vi "Main.vi"() -> ()   [LabVIEW 2022 SP3]
uses:
  Controls/MainStates.ctl
  <userlib>/_OpenG.lib/array/array.llb/Remove Duplicates from 1D Array (String)__ogtk.vi
panel:
  in  "Clean after \"(\"":bool
  out "New":string
  out "Old":string
  out "new path":path
  in  "Auto":enum32{"Manual", "MKV", "AVI", "MP4", "MP3"}(radio)
  in  "Commit":bool
  in  "Replacement String":string
  in  "Split Key":string="("
  in  "Method":T1(ring)
  in  "Extension":string=".*"
  in  "Path":path
  out "New":i32(listbox)
  out "Current":i32(listbox)=1
  in  "Exit":bool
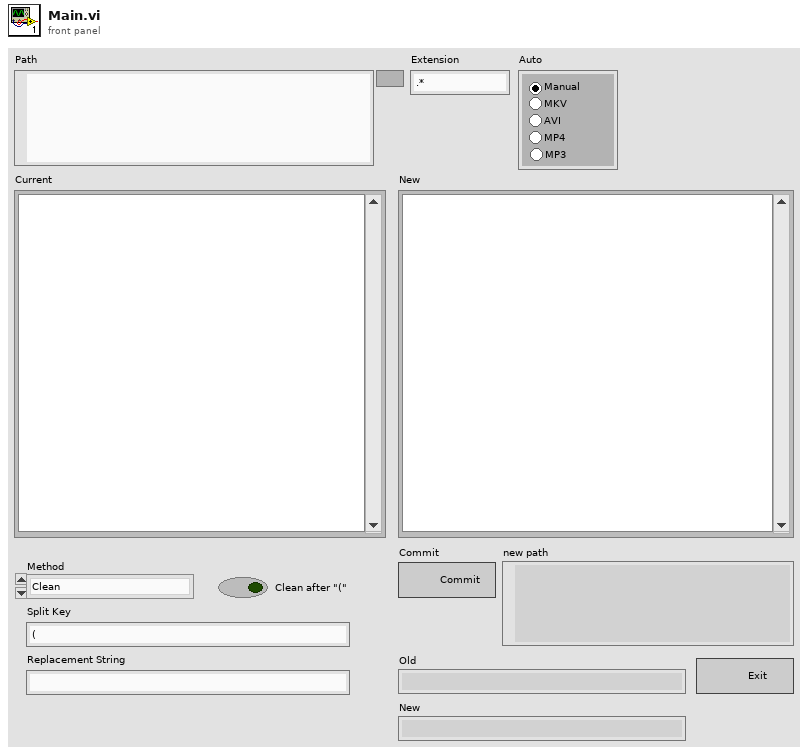
[diagram p1: front panel]
types:
  T1 = enum16{"Clean", "Replace", "Clear Periods", "Strip Prefix", "Add Prefix"}
  T2 = typedef "MainStates.ctl" = enum16{"Init", "Get Path", "Get Files", "Set Extension", "Check for Dups", "Clean", "Add Prefix", "Replace", "Periods", "Strip Prefix", "Commit", "Wait for Input", "Exit"}
  T3 = enum8{"Enabled", "Disabled", "Disabled and Grayed Out"}
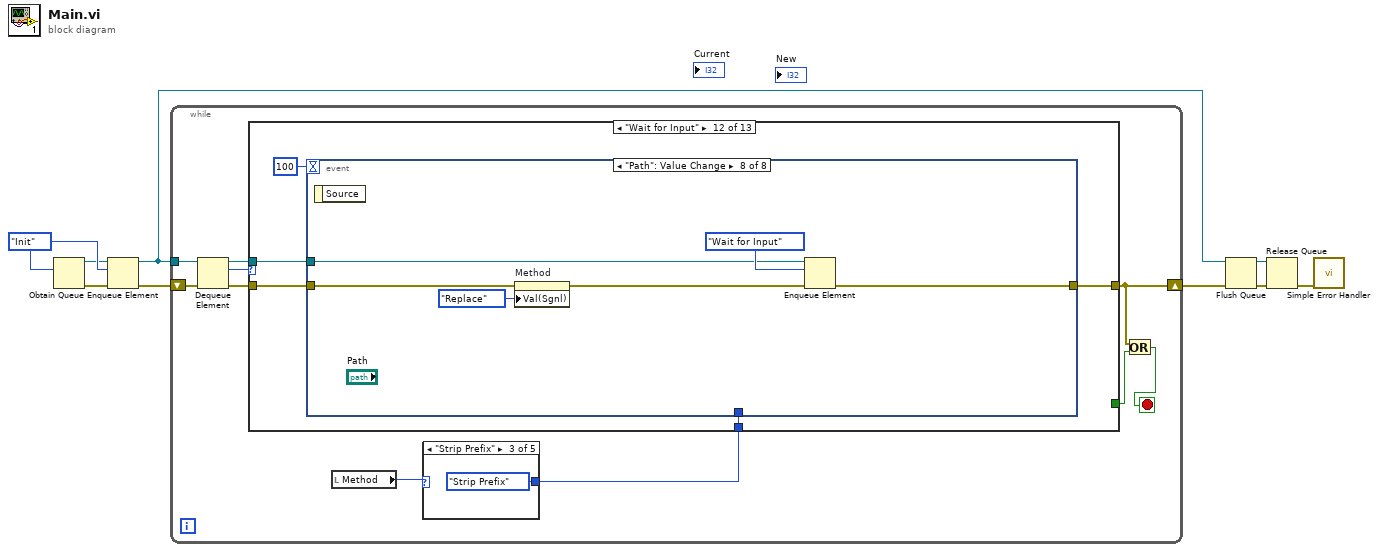
[diagram p0: block diagram]
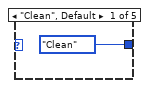
[diagram p2: hidden frame]
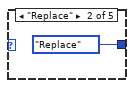
[diagram p3: hidden frame]
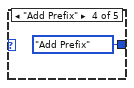
[diagram p4: hidden frame]
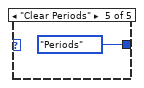
[diagram p5: hidden frame]
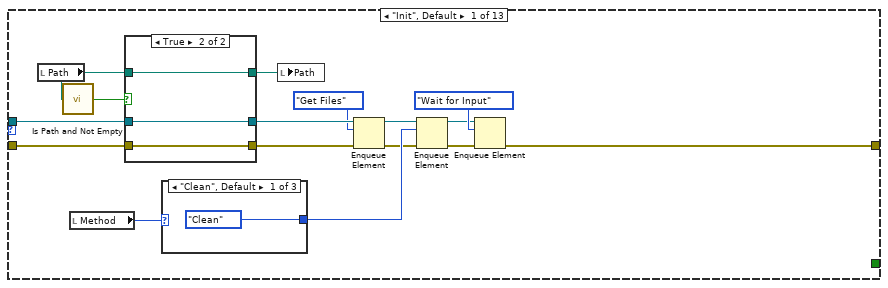
[diagram p6: hidden frame]
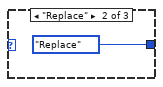
[diagram p7: hidden frame]
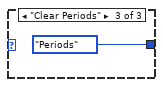
[diagram p8: hidden frame]
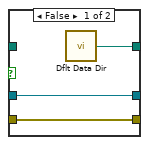
[diagram p9: hidden frame]
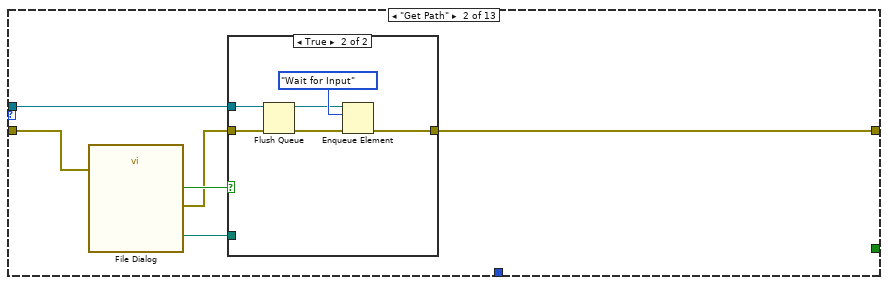
[diagram p10: hidden frame]
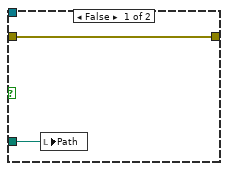
[diagram p11: hidden frame]
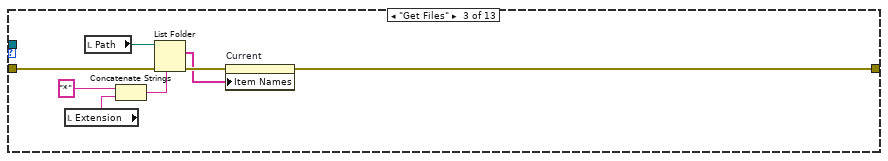
[diagram p12: hidden frame]
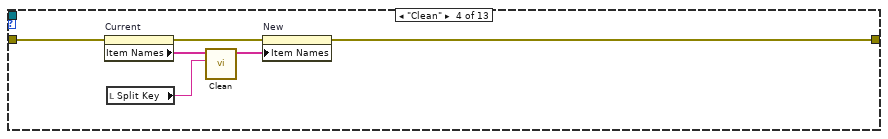
[diagram p13: hidden frame]
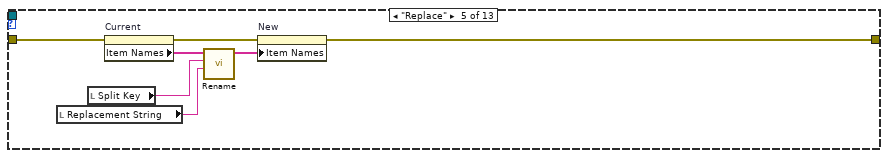
[diagram p14: hidden frame]
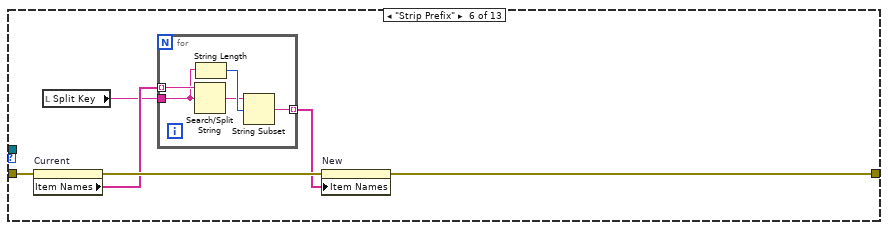
[diagram p15: hidden frame]
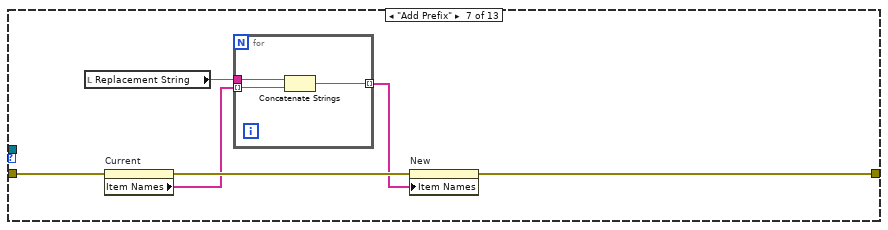
[diagram p16: hidden frame]
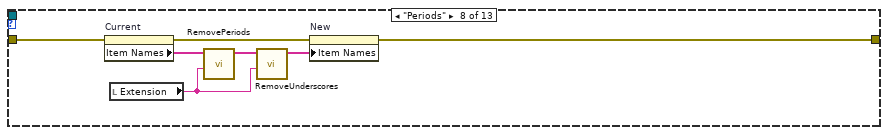
[diagram p17: hidden frame]
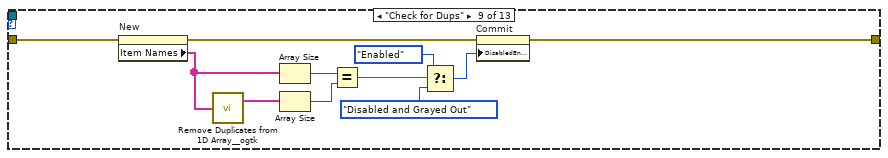
[diagram p18: hidden frame]
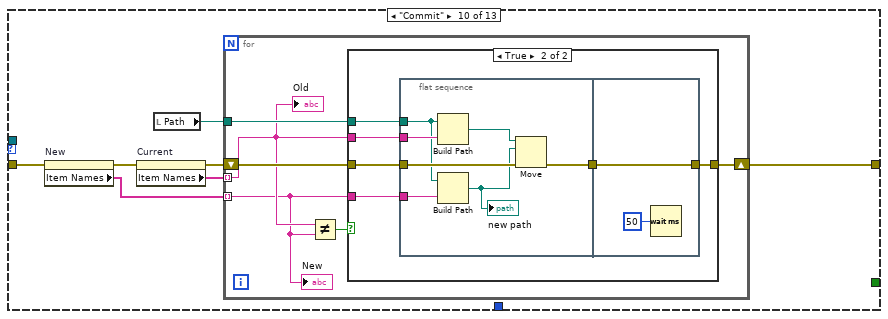
[diagram p19: hidden frame]
diagram:
  w9 = MainStates."Init" ("Main States")
  n1 = Obtain Queue(element data type=w9) -> (queue out=w8:refnum<queue>, error out=w7:errorcluster)  [unwired: 4 in, 1 out]
  n2 = Enqueue Element(queue=w8, element=w9, error in (no error)=w7) -> (queue out=w4:refnum<queue>, error out=w6:errorcluster)  [unwired: 1 in, 1 out]
  n3 = while {
    tunnel: w4 -> [w18]
    shift-right: [w12] -> w3
    shift-left: w6 -> [w19]
    stop <- w10 stop-if-true
    n4 = Dequeue Element(queue=w18, error in (no error)=w19) -> (queue out=w16:refnum<queue>, element=w17:T2, error out=w15:errorcluster)  [unwired: 1 in, 1 out]
    n5 = local read "Method"() -> (w14:T1)
    n6 = case shown="\"Strip Prefix\"" w14 {
      tunnel: [MainStates."Clean" ("Main States") MainStates."Replace" ("Main States") MainStates."Strip Prefix" ("Main States") MainStates."Add Prefix" ("Main States") MainStates."Periods" ("Main States")] -> w13
      frame "Clean", Default {
      }
      frame "Replace" {
      }
      frame "Strip Prefix" {
      }
      frame "Add Prefix" {
      }
      frame "Clear Periods" {
      }
    }
    n7 = case shown="\"Wait for Input\"" w17 {
      tunnel: w16 -> [w36 w53 _ _ _ _ _ _ _ _ _ w165 _]
      tunnel: w15 -> [w37 w55 w70 w77 w84 w90 w101 w111 w122 w127 w154 w164 w238]
      tunnel: [w39 w51 w64 w72 w78 w88 w99 w108 w115 w123 w152 w163 w238] -> w12
      tunnel: [_ _ _ _ _ _ _ _ _ _ _ _ TRUE] -> w11
      tunnel: w13 -> [_ _ _ _ _ _ _ _ _ _ _ w162 _]
      frame "Init", Default {
        n8 = local read "Path"() -> (w26:path)
        n9 = call <vilib>:"Is Path and Not Empty.vi"("path"=w26) -> ("Is Path and Not Empty?"=w38:bool)  [unwired: 4 in]
        n10 = local read "Method"() -> (w33:T1)
        n11 = case shown="True" w38 {
          tunnel: w37 -> [w45 w48]
          tunnel: w36 -> [w46 w49]
          tunnel: [w46 w49] -> w35
          tunnel: [w45 w48] -> w34
          tunnel: w26 -> [_ w47]
          tunnel: [w44 w47] -> w25
          frame False {
            n12 = call <vilib>:"Dflt Data Dir.vi"() -> ("App:Default Data Directory"=w44:path)
          }
          frame True {
          }
        }
        n13 = case shown="\"Clean\", Default" w33 {
          tunnel: [MainStates."Clean" ("Main States") MainStates."Replace" ("Main States") MainStates."Periods" ("Main States")] -> w30
          frame "Clean", Default {
          }
          frame "Replace" {
          }
          frame "Clear Periods" {
          }
        }
        n14 = local write "Path"(w25) -> ()
        n15 = Enqueue Element(queue=w35, element=MainStates."Get Files" ("Main States"), error in (no error)=w34) -> (queue out=w28:refnum<queue>, error out=w27:errorcluster)  [unwired: 1 in, 1 out]
        n16 = Enqueue Element(queue=w28, element=w30, error in (no error)=w27) -> (queue out=w31:refnum<queue>, error out=w32:errorcluster)  [unwired: 1 in, 1 out]
        n17 = Enqueue Element(queue=w31, element=MainStates."Wait for Input" ("Main States"), error in (no error)=w32) -> (error out=w39:errorcluster)  [unwired: 1 in, 2 out]
      }
      frame "Get Path" {
        n18 = call "File Dialog"("error in"=w55) -> ("selected path"=w50:path, "cancelled"=w54:bool, "error out"=w52:errorcluster)  [unwired: 11 in, 1 out]
        n19 = case shown="True" w54 {
          tunnel: w53 -> [_ w63]
          tunnel: w52 -> [w56 w62]
          tunnel: [w56 w58] -> w51
          tunnel: w50 -> [w57 _]
          frame False {
            n20 = local write "Path"(w57) -> ()
          }
          frame True {
            n21 = Flush Queue(queue=w63, error in (no error)=w62) -> (queue out=w60:refnum<queue>, error out=w59:errorcluster)  [unwired: 1 out]
            n22 = Enqueue Element(queue=w60, element=MainStates."Wait for Input" ("Main States"), error in (no error)=w59) -> (error out=w58:errorcluster)  [unwired: 1 in, 2 out]
          }
        }
      }
      frame "Get Files" {
        n23 = local read "Extension"() -> (w65:string)
        n24 = local read "Path"() -> (w71:path)
        n25 = Concatenate Strings("*", w65) -> (w66:string)
        n26 = List Folder(path=w71, pattern=w66, error in=w70) -> (filenames=w68:string[], error out=w69:errorcluster)  [unwired: 1 in, 2 out]
        n27 = property on="Current" class="LstBox (strict)"(error in=w69, "Item Names"=w68) -> (error out=w64:errorcluster)  [unwired: 1 in, 1 out]
      }
      frame "Clean" {
        n28 = property on="Current" class="LstBox (strict)"(error in=w77) -> (error out=w73:errorcluster, "Item Names"=w76:string[])  [unwired: 1 in, 1 out]
        n29 = local read "Split Key"() -> (w75:string)
        n30 = call "Clean.vi"("Split Key"=w75, "Filenames In"=w76) -> ("Filenames Out"=w74:string[])  [unwired: 9 in]
        n31 = property on="New" class="LstBox (strict)"(error in=w73, "Item Names"=w74) -> (error out=w72:errorcluster)  [unwired: 1 in, 1 out]
      }
      frame "Replace" {
        n32 = local read "Replacement String"() -> (w81:string)
        n33 = local read "Split Key"() -> (w82:string)
        n34 = property on="Current" class="LstBox (strict)"(error in=w84) -> (error out=w79:errorcluster, "Item Names"=w83:string[])  [unwired: 1 in, 1 out]
        n35 = call "Rename.vi"("Replacement String"=w81, "Split Key"=w82, "Filenames In"=w83) -> ("Filenames Out"=w80:string[])  [unwired: 8 in]
        n36 = property on="New" class="LstBox (strict)"(error in=w79, "Item Names"=w80) -> (error out=w78:errorcluster)  [unwired: 1 in, 1 out]
      }
      frame "Strip Prefix" {
        n37 = property on="Current" class="LstBox (strict)"(error in=w90) -> (error out=w89:errorcluster, "Item Names"=w87:string[])  [unwired: 1 in, 1 out]
        n38 = local read "Split Key"() -> (w86:string)
        n39 = for {
          tunnel: w87 -> [w95] mode=indexing
          tunnel: w86 -> [w94]
          tunnel: [w91] -> w85 mode=indexing
          n40 = Search/Split String(string=w95, search string/char (-)=w94) -> (match + rest of string=w92:string)  [unwired: 1 in, 2 out]
          n41 = String Length(string=w94) -> (length=w93:i32)
          n42 = String Subset(string=w92, offset (0)=w93) -> (substring=w91:string)  [unwired: 1 in]
        }
        n43 = property on="New" class="LstBox (strict)"(error in=w89, "Item Names"=w85) -> (error out=w88:errorcluster)  [unwired: 1 in, 1 out]
      }
      frame "Add Prefix" {
        n44 = local read "Replacement String"() -> (w97:string)
        n45 = property on="Current" class="LstBox (strict)"(error in=w101) -> (error out=w100:errorcluster, "Item Names"=w98:string[])  [unwired: 1 in, 1 out]
        n46 = for {
          tunnel: w98 -> [w104] mode=indexing
          tunnel: w97 -> [w103]
          tunnel: [w102] -> w96 mode=indexing
          n47 = Concatenate Strings(w103, w104) -> (w102:string)
        }
        n48 = property on="New" class="LstBox (strict)"(error in=w100, "Item Names"=w96) -> (error out=w99:errorcluster)  [unwired: 1 in, 1 out]
      }
      frame "Periods" {
        n49 = property on="Current" class="LstBox (strict)"(error in=w111) -> (error out=w109:errorcluster, "Item Names"=w110:string[])  [unwired: 1 in, 1 out]
        n50 = local read "Extension"() -> (w105:string)
        n51 = call "RemovePeriods.vi"("Extension"=w105, "Filenames In"=w110) -> ("Filenames Out"=w107:string[])  [unwired: 9 in]
        n52 = call "RemoveUnderscores.vi"("Extension"=w105, "Filenames In"=w107) -> ("Filenames Out"=w106:string[])  [unwired: 9 in]
        n53 = property on="New" class="LstBox (strict)"(error in=w109, "Item Names"=w106) -> (error out=w108:errorcluster)  [unwired: 1 in, 1 out]
      }
      frame "Check for Dups" {
        n54 = property on="New" class="LstBox (strict)"(error in=w122) -> (error out=w116:errorcluster, "Item Names"=w121:string[])  [unwired: 1 in, 1 out]
        n55 = call-poly <userlib>:"Remove Duplicates from 1D Array__ogtk.vi"("Input Array"=w121) -> ("Output Array"=w120:string[])  [unwired: 1 out]
        n56 = Array Size(array=w121) -> (size(s)=w119:i32)
        n57 = Array Size(array=w120) -> (size(s)=w118:i32)
        n58 = Equal?(x=w119, y=w118) -> (x = y?=w117:bool)
        n59 = Select(t=T3."Enabled" ("Disabled"), s=w117, f=T3."Disabled and Grayed Out" ("Disabled")) -> (s? t:f=w112:T3)
        n60 = property on="Commit" class="Bool"(error in=w116, "DisabledEnum"=w112) -> (error out=w115:errorcluster)  [unwired: 1 in, 1 out]
      }
      frame "Commit" {
        n61 = property on="New" class="LstBox (strict)"(error in=w127) -> (error out=w126:errorcluster, "Item Names"=w125:string[])  [unwired: 1 in, 1 out]
        n62 = property on="Current" class="LstBox (strict)"(error in=w126) -> (error out=w124:errorcluster, "Item Names"=w128:string[])  [unwired: 1 in, 1 out]
        n63 = local read "Path"() -> (w129:path)
        n64 = for {
          tunnel: w129 -> [w134]
          tunnel: w128 -> [w131] mode=indexing
          tunnel: w125 -> [w130] mode=indexing
          shift-right: [w133] -> w123
          shift-left: w124 -> [w135]
          n65 = Not Equal?(x=w131, y=w130) -> (x != y?=w132:bool)
          n66 = case shown="True" w132 {
            tunnel: w131 -> [_ w142]
            tunnel: w135 -> [w136 w141]
            tunnel: w134 -> [_ w140]
            tunnel: w130 -> [_ w139]
            tunnel: [w136 w138] -> w133
            frame False {
            }
            frame True {
              n67 = flat-sequence {
                tunnel: w142 -> [w149]
                tunnel: w141 -> [w148]
                tunnel: w140 -> [w147]
                tunnel: w139 -> [w146]
                tunnel: [w143] -> w137
                tunnel: [w151] -> w138
                tunnel: w137 -> [w151]
                frame #0 {
                  n68 = Build Path(base path=w147, name or relative path=w149) -> (appended path=w145:path)
                  n69 = Build Path(base path=w147, name or relative path=w146) -> (appended path=w144:path)
                  "new path" <- w144
                  n70 = Move(source path=w145, error in=w148, 10:w144) -> (error out=w143:errorcluster)  [unwired: 2 in, 2 out]
                }
                frame #1 {
                  n71 = Wait (ms)(milliseconds to wait=u32 50) -> ()  [unwired: 1 out]
                }
              }
            }
          }
          "Old" <- w131
          "New" <- w130
        }
      }
      frame "Set Extension" {
        n72 = local read "Auto"() -> (w155:enum32{"Manual", "MKV", "AVI", "MP4", "MP3"})
        n73 = case shown="\"MP3\"" w155 {
          tunnel: [".*" ".mkv" ".avi" ".mp4" ".mp3"] -> w153
          frame "Manual", Default {
          }
          frame "MKV" {
          }
          frame "AVI" {
          }
          frame "MP4" {
          }
          frame "MP3" {
          }
        }
        n74 = property on="Extension" class="Str"(error in=w154, "Val(Sgnl)"=w153) -> (error out=w152:errorcluster)  [unwired: 1 in, 1 out]
      }
      frame "Wait for Input" {
        n75 = event shown="[7] \"Path\": Value Change" {
          selector: _ -> [_ _ _ _ _ _ _ _]
          dyn-events: _ -> [_ _ _ _ _ _ _ _]
          timeout: 100 -> [_ _ _ _ _ _ _ _]
          tunnel: w165 -> [w169 w181 w188 w204 w217 w225 w229 w235]
          tunnel: w164 -> [w168 w180 w189 w205 w216 w223 w228 w234]
          tunnel: [w167 w178 w183 w197 w214 w219 w230 w236] -> w163
          tunnel: w162 -> [_ w177 _ w196 w212 _ _ _]
          event "Exit": Value Change {
            n76 = event-data() -> ()  [unwired: 1 in, 1 out]
            n77 = Enqueue Element(queue=w169, element=MainStates."Exit" ("Main States"), error in (no error)=w168) -> (error out=w167:errorcluster)  [unwired: 1 in, 2 out]
          }
          event Timeout {
            n78 = event-data() -> ()  [unwired: 1 in, 3 out]
            n79 = Enqueue Element(queue=w181, element=MainStates."Get Files" ("Main States"), error in (no error)=w180) -> (queue out=w175:refnum<queue>, error out=w174:errorcluster)  [unwired: 1 in, 1 out]
            n80 = Enqueue Element(queue=w175, element=w177, error in (no error)=w174) -> (queue out=w173:refnum<queue>, error out=w172:errorcluster)  [unwired: 1 in, 1 out]
            n81 = Enqueue Element(queue=w173, element=MainStates."Check for Dups" ("Main States"), error in (no error)=w172) -> (queue out=w171:refnum<queue>, error out=w170:errorcluster)  [unwired: 1 in, 1 out]
            n82 = Enqueue Element(queue=w171, element=MainStates."Wait for Input" ("Main States"), error in (no error)=w170) -> (error out=w178:errorcluster)  [unwired: 1 in, 2 out]
          }
          event "Method", "Replacement String", "Split Key": Value Change {
            n83 = event-data() -> ()  [unwired: 1 in, 1 out]
            n84 = case shown="\"Clean\", Default" "Method" {
              tunnel: [MainStates."Clean" ("Main States") MainStates."Replace" ("Main States") MainStates."Strip Prefix" ("Main States") MainStates."Add Prefix" ("Main States") MainStates."Periods" ("Main States")] -> w187
              frame "Clean", Default {
              }
              frame "Replace" {
              }
              frame "Strip Prefix" {
              }
              frame "Add Prefix" {
              }
              frame "Clear Periods" {
              }
            }
            n85 = Enqueue Element(queue=w188, element=w187, error in (no error)=w189) -> (queue out=w184:refnum<queue>, error out=w185:errorcluster)  [unwired: 1 in, 1 out]
            n86 = Enqueue Element(queue=w184, element=MainStates."Wait for Input" ("Main States"), error in (no error)=w185) -> (error out=w183:errorcluster)  [unwired: 1 in, 2 out]
          }
          event "Extension": Value Change {
            n87 = event-data() -> ()  [unwired: 1 in, 1 out]
            n88 = Enqueue Element(queue=w204, element=MainStates."Get Files" ("Main States"), error in (no error)=w205) -> (queue out=w201:refnum<queue>, error out=w202:errorcluster)  [unwired: 1 in, 1 out]
            n89 = Enqueue Element(queue=w201, element=w196, error in (no error)=w202) -> (queue out=w199:refnum<queue>, error out=w198:errorcluster)  [unwired: 1 in, 1 out]
            n90 = Enqueue Element(queue=w199, element=MainStates."Wait for Input" ("Main States"), error in (no error)=w198) -> (error out=w197:errorcluster)  [unwired: 1 in, 2 out]
          }
          event "Commit": Value Change {
            n91 = event-data() -> ()  [unwired: 1 in, 1 out]
            n92 = Enqueue Element(queue=w217, element=MainStates."Commit" ("Main States"), error in (no error)=w216) -> (queue out=w210:refnum<queue>, error out=w211:errorcluster)  [unwired: 1 in, 1 out]
            n93 = Enqueue Element(queue=w210, element=MainStates."Get Files" ("Main States"), error in (no error)=w211) -> (queue out=w209:refnum<queue>, error out=w208:errorcluster)  [unwired: 1 in, 1 out]
            n94 = Enqueue Element(queue=w209, element=w212, error in (no error)=w208) -> (queue out=w206:refnum<queue>, error out=w207:errorcluster)  [unwired: 1 in, 1 out]
            n95 = Enqueue Element(queue=w206, element=MainStates."Wait for Input" ("Main States"), error in (no error)=w207) -> (error out=w214:errorcluster)  [unwired: 1 in, 2 out]
          }
          event "Auto": Value Change {
            n96 = event-data() -> ()  [unwired: 1 in, 1 out]
            n97 = Enqueue Element(queue=w225, element=MainStates."Set Extension" ("Main States"), error in (no error)=w223) -> (queue out=w220:refnum<queue>, error out=w221:errorcluster)  [unwired: 1 in, 1 out]
            n98 = Enqueue Element(queue=w220, element=MainStates."Wait for Input" ("Main States"), error in (no error)=w221) -> (error out=w219:errorcluster)  [unwired: 1 in, 2 out]
          }
          event "Clean after \"(\"": Value Change {
            n99 = event-data() -> ()  [unwired: 1 in, 1 out]
            n100 = property on="Split Key" class="Str"(error in=w228, "Val(Sgnl)"="(" ("Split Key")) -> (error out=w227:errorcluster)  [unwired: 1 in, 1 out]
            n101 = Enqueue Element(queue=w229, element=MainStates."Wait for Input" ("Main States"), error in (no error)=w227) -> (error out=w230:errorcluster)  [unwired: 1 in, 2 out]
          }
          event "Path": Value Change {
            n102 = event-data() -> ()  [unwired: 1 in, 1 out]
            n103 = property on="Method" class="Enum (strict)"(error in=w234, "Val(Sgnl)"=T1."Replace" ("Value (Signaling)")) -> (error out=w233:errorcluster)  [unwired: 1 in, 1 out]
            n104 = Enqueue Element(queue=w235, element=MainStates."Wait for Input" ("Main States"), error in (no error)=w233) -> (error out=w236:errorcluster)  [unwired: 1 in, 2 out]
          }
        }
      }
      frame "Exit" {
      }
    }
    n105 = Or(x=w12, y=w11) -> (x .or. y?=w10:bool)
  }
  n106 = Flush Queue(queue=w4, error in (no error)=w3) -> (queue out=w1:refnum<queue>, error out=w5:errorcluster)  [unwired: 1 out]
  n107 = Release Queue(queue=w1, error in (no error)=w5) -> (error out=w2:errorcluster)  [unwired: 1 in, 2 out]
  n108 = call <vilib>:"Simple Error Handler.vi"("error in (no error)"=w2) -> ()  [unwired: 4 in, 5 out]
